vi "lv_icon.vi"(8 "error in (no error)":errorcluster, 9 "BW icon in":T1, 10 "Color icon in":T1, 11 "_Class 4 in":refnum<class "Class 4.lvclass">) -> (0 "error out":errorcluster, 1 "Color icon out":T1, 2 "BW icon out":T1, 3 "_Class 4 out":refnum<class "Class 4.lvclass">, 4 "Error code out":i32)   [LabVIEW 2021, in "Class 4.lvclass"]
uses:
  Class 4.lvclass
  Class 4.lvclass/Class 4.ctl
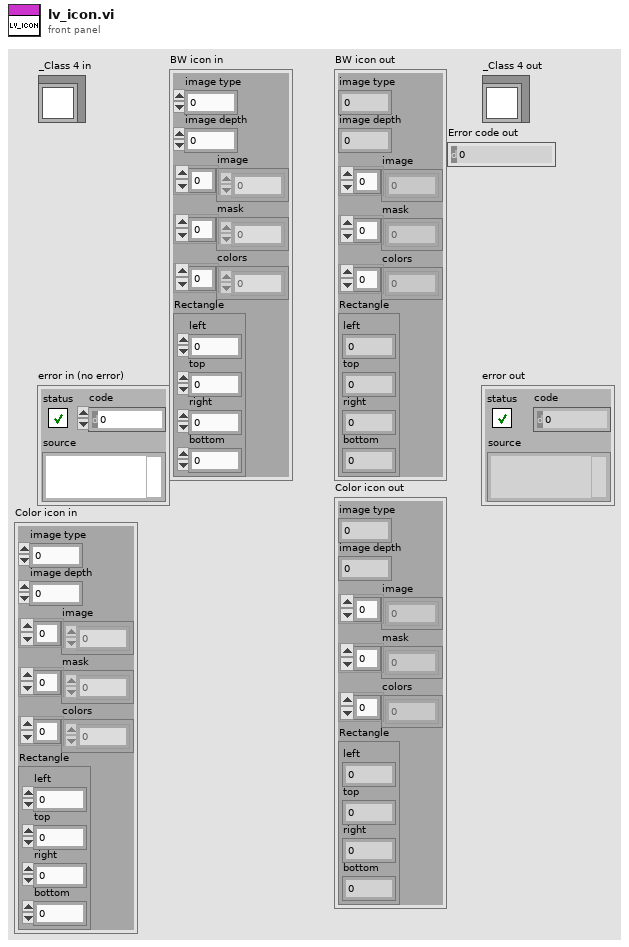
[diagram p1: front panel]
types:
  T1 = cluster{"image type":i32, "image depth":i32, "image":u8[], "mask":u8[], "colors":u32[], "Rectangle":cluster{"left":i16, "top":i16, "right":i16, "bottom":i16}}
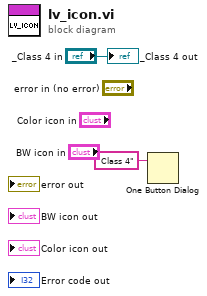
[diagram p0: block diagram]
diagram:
  n1 = One Button Dialog(message="Class 4") -> ()  [unwired: 1 in, 1 out]
  "_Class 4 out" <- "_Class 4 in"
